vi "Autonomous Independent.vi"() -> ()   [LabVIEW 2013]
doc: "This VI is called when autonomous begins, and will automatically be terminated when autonomous ends. You can carry out timed or sensor driven robot movement independently without needing to return to the caller."
uses:
  Robot Global Data.vi
  <vilib>/addons/control/pid/pid.llb/PID (DBL).vi
  <vilib>/Rock Robotics/WPI/Joystick/WPI_JoystickGetSetRefNum.vi
  <vilib>/addons/control/pid/NI_PID_pid.lvlib
panel:
  out "Driver Station Digital Input (1-8)":bool[](array[boolean])
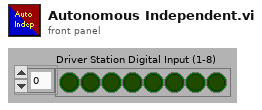
[diagram p1: front panel]
types:
  T1 = typedef "WPI_JoystickDevRef.ctl" = cluster{"Device":T2}
  T2 = typedef "WPI_JoystickDeviceEnum.ctl" = enum16{"USB 1", "USB 2", "USB 3", "USB 4", "Kinect 1", "Kinect 2"}
  T3 = cluster{"axis 1 (x)":dbl, "axis 2 (y)":dbl, "axis 3 (throttle)":dbl, "axis 4":dbl, "axis 5":dbl, "axis 6":dbl}
  T4 = cluster{"Driver Station Digital Input (1-8)[0]":bool, "Driver Station Digital Input (1-8)[1]":bool, "Driver Station Digital Input (1-8)[2]":bool, "Driver Station Digital Input (1-8)[3]":bool, "Driver Station Digital Input (1-8)[4]":bool, "Driver Station Digital Input (1-8)[5]":bool, "Driver Station Digital Input (1-8)[6]":bool, "Driver Station Digital Input (1-8)[7]":bool, "Driver Station Digital Input (1-8)[8]":bool}
  T5 = cluster{"proportional gain (Kc)":dbl, "integral time (Ti, min)":dbl, "derivative time (Td, min)":dbl}
  T6 = typedef "WPI_MotorControlDeviceRef.ctl" = cluster{"DeviceStatus":errorcluster, "Type":enum16{"PWM", "CAN"}, "PWM":cluster{"Digital Module":T7, "PWM Channel":T8, "DeadBand":T9}, "CAN":cluster{"Device Number":u8, "Control Mode":T10, "Semaphore":T11, "Max Vout":dbl}, "Invert":bool, "TransformRef":T12, "InvTransformRef":T12}
  T7 = typedef "FPGA_TypedefDigitalModule.ctl" = enum16{"Digital Module 1", "Digital Module 2"}
  T8 = typedef "FPGA_DIOPWMChannel.ctl" = enum8{"PWM 1", "PWM 2", "PWM 3", "PWM 4", "PWM 5", "PWM 6", "PWM 7", "PWM 8", "PWM 9", "PWM 10", "Invalid"}
  T9 = typedef "WPI_PWMDeadband.ctl" = cluster{"Name":string, "maxPositivePwm":i32, "minPositivePwm":i32, "centerPwm":i32, "maxNegativePwm":i32, "minNegativePwm":i32, "angularRange":u16}
  T10 = typedef "WPI_CANJaguar_ControlMode.ctl" = enum8{"Percent VBus", "Current", "Speed", "Position", "Voltage"}
  T11 = typedef "Semaphore RefNum" = refnum<k1>
  T12 = typedef "WPI_PWMTransform_ConPane.ctl" = refnum<vi>
  T13 = typedef "WPI_RobotDriveDevRef.ctl" = cluster{"DevStatus":errorcluster, "Motors[]":T6[], "Square Inputs":bool, "Max Output":dbl, "Isochronous":bool}
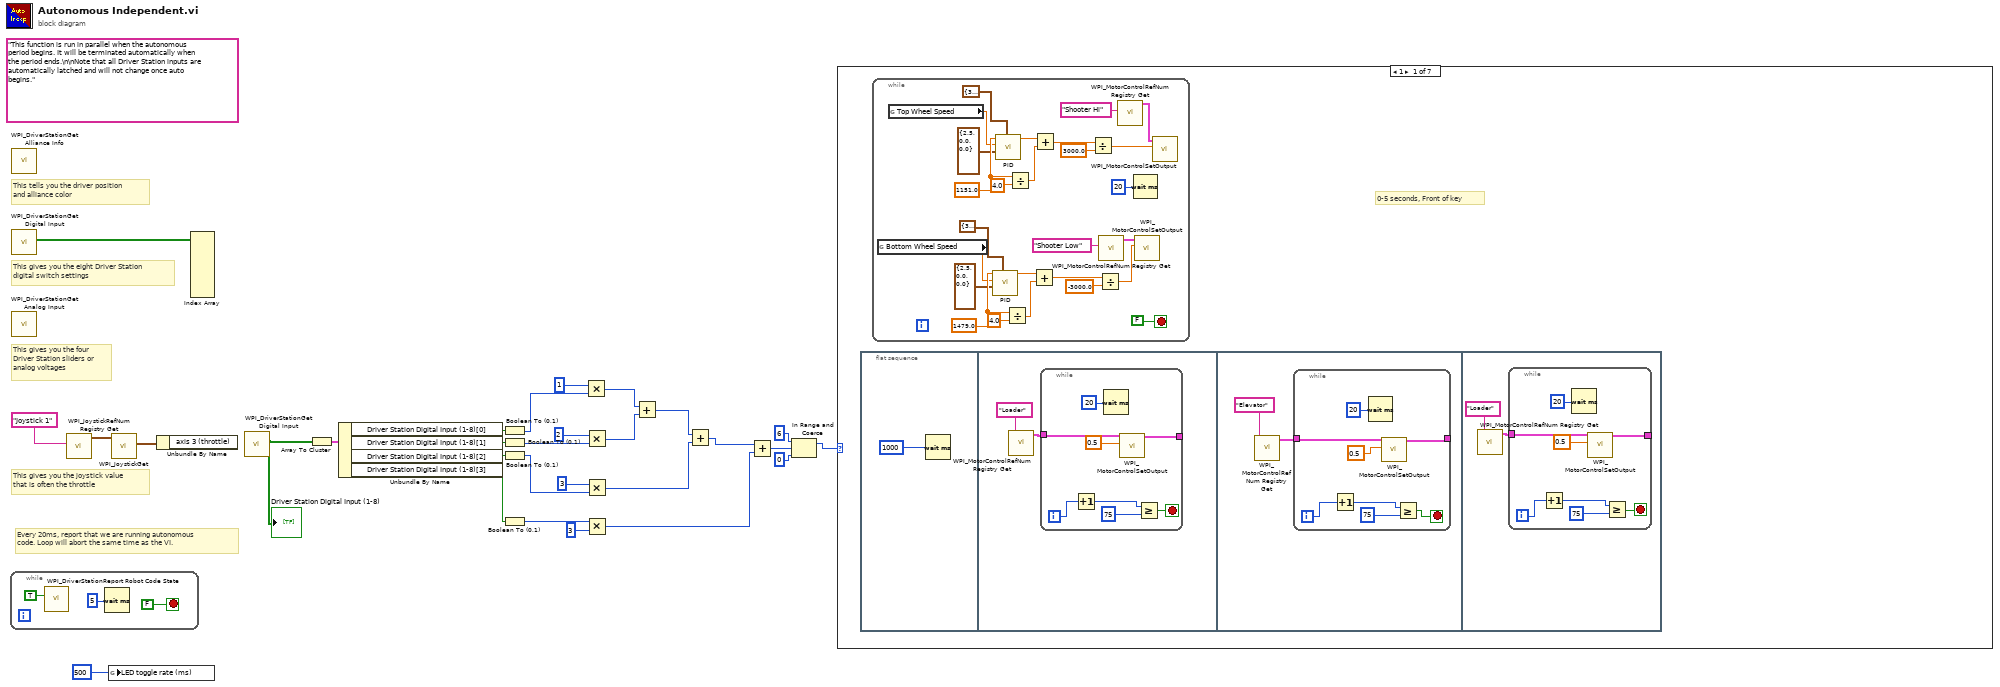
[diagram p0: block diagram]
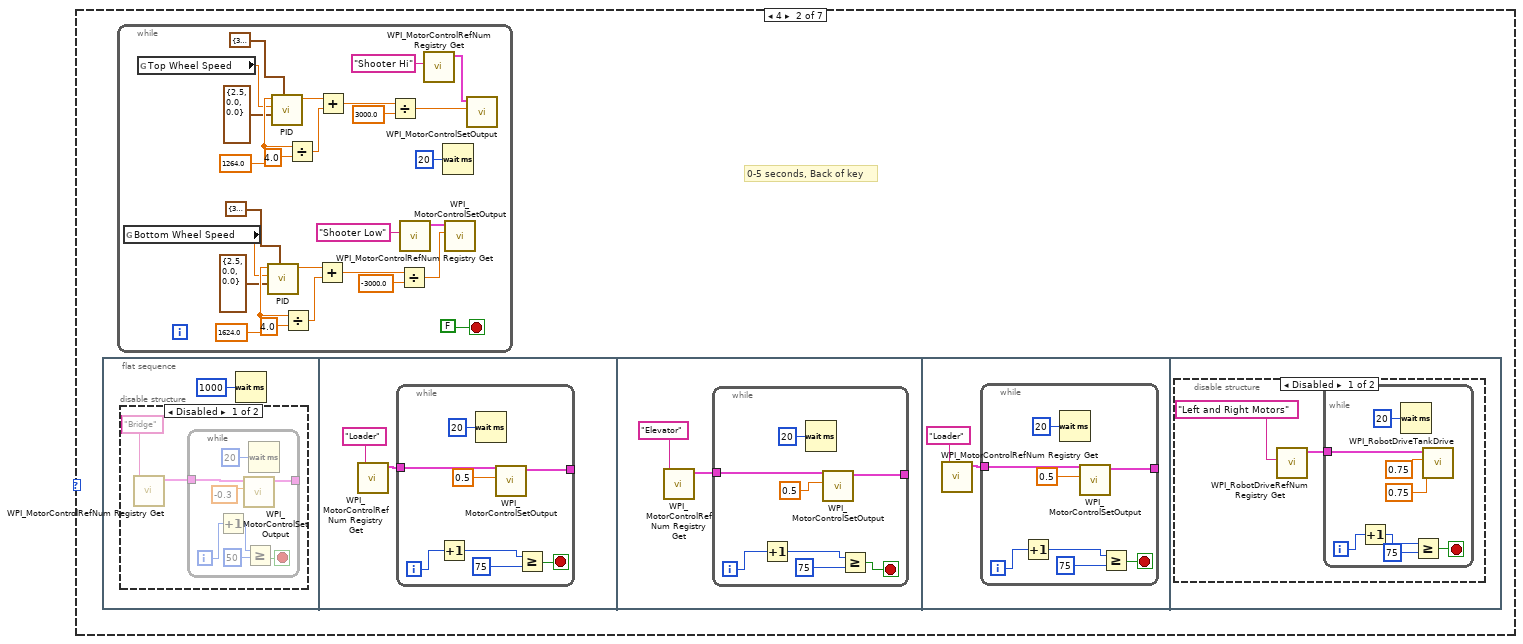
[diagram p2: hidden frame]
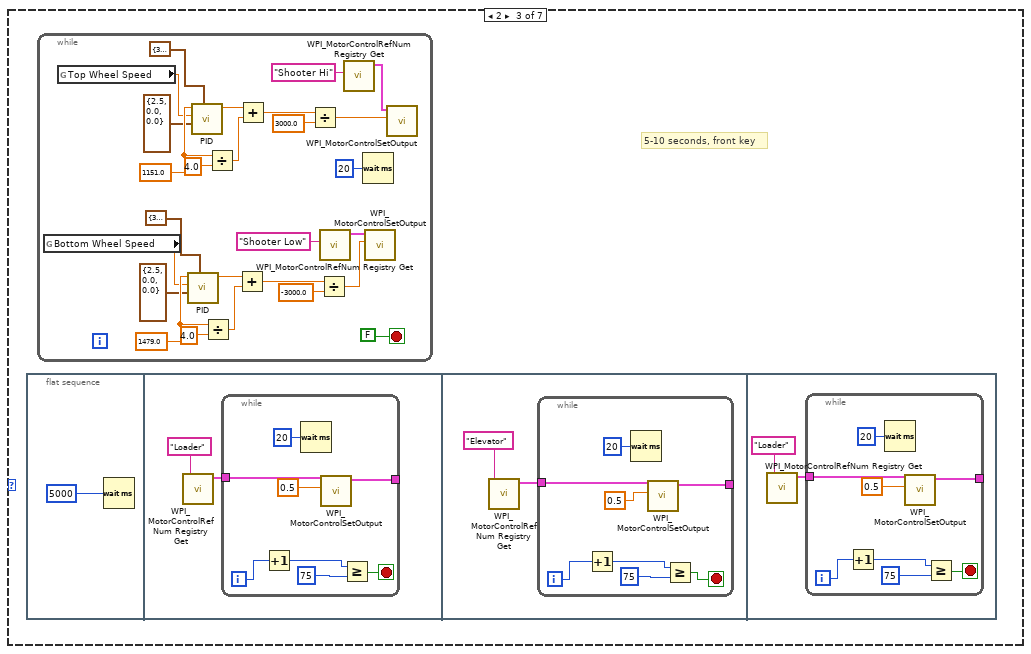
[diagram p5: hidden frame]
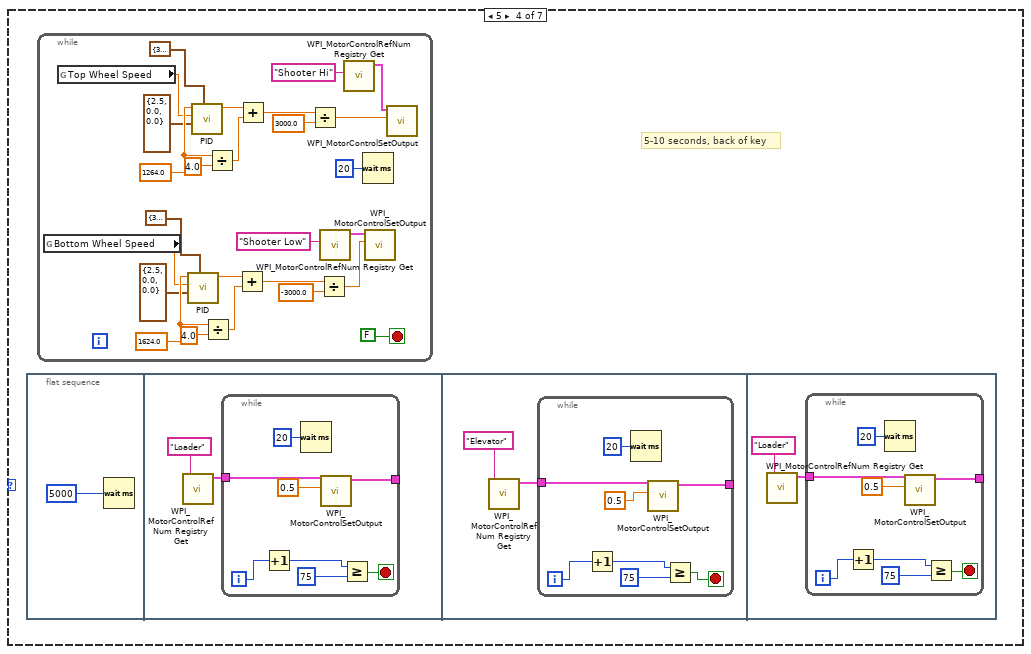
[diagram p6: hidden frame]
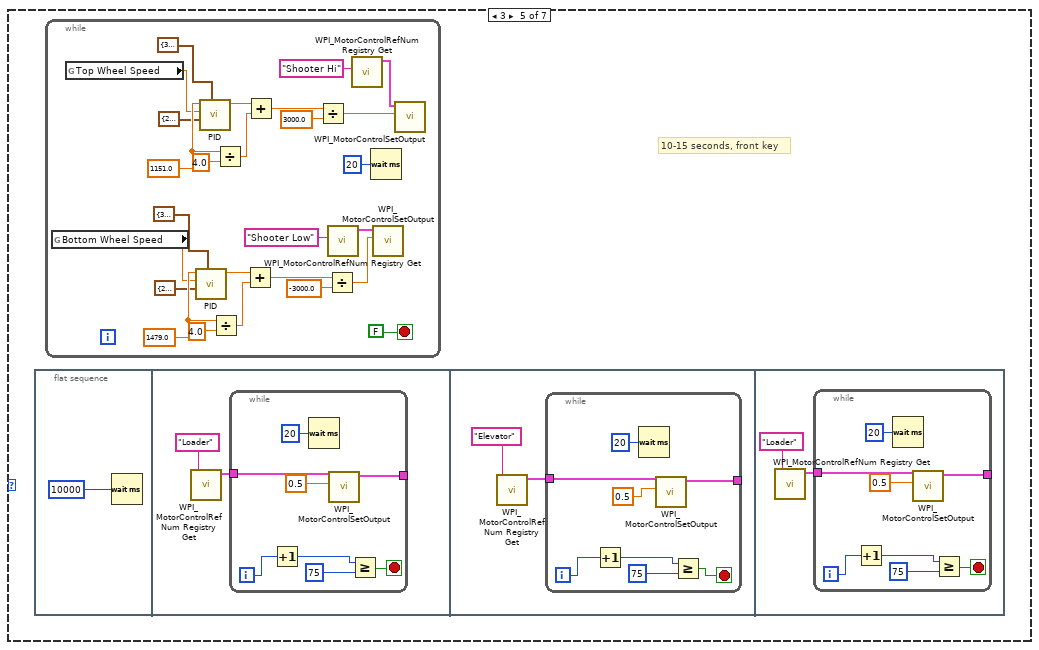
[diagram p7: hidden frame]
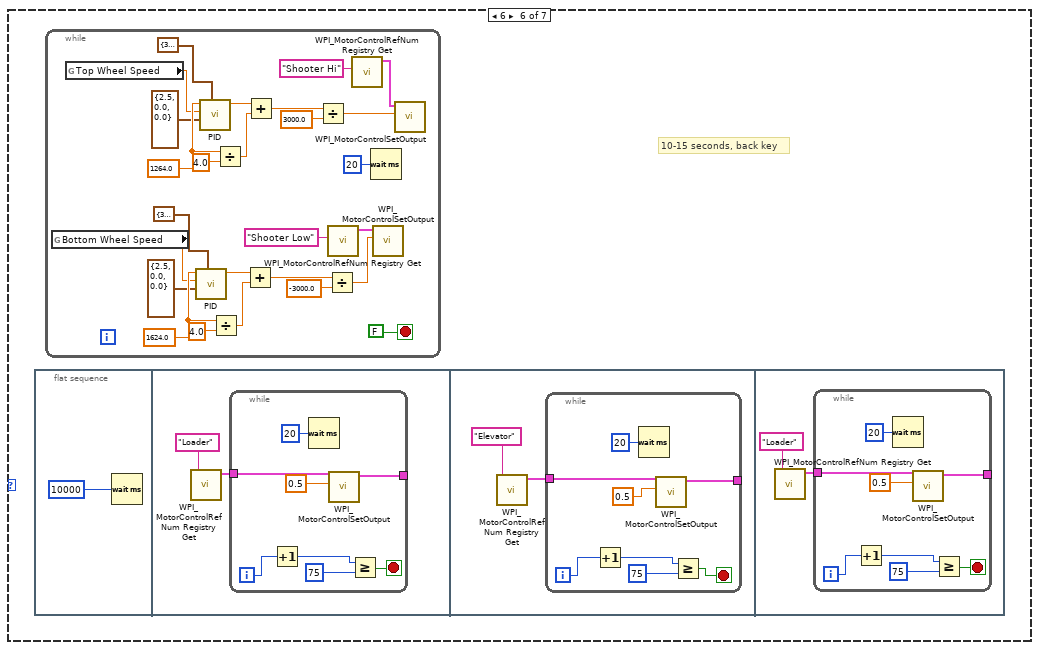
[diagram p8: hidden frame]
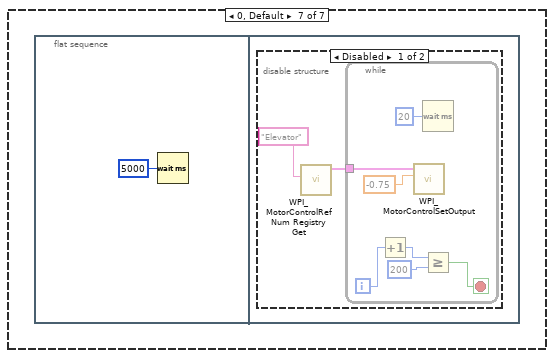
[diagram p9: hidden frame]
diagram:
  (unwired) "This function is run in parallel when the autonomous period begins. It will be terminated automatically when the period ends.\n\nNote that all Driver Station inputs are automatically latched and will not change once auto begins."
  # "Every 20ms, report that we are running autonomous\ncode. Loop will abort the same time as the VI."
  # "This gives you the joystick value\nthat is often the throttle"
  # "This tells you the driver position\nand alliance color"
  # "This gives you the eight Driver Station\ndigital switch settings"
  # "This gives you the four\nDriver Station sliders or\nanalog voltages"
  n1 = while {
    stop <- FALSE stop-if-true
    n2 = call <vilib>:"WPI_DriverStationReport Robot Code State.vi"("Autonomous"=TRUE) -> ()  [unwired: 10 in, 1 out]
    n3 = Wait (ms)(milliseconds to wait=u32 5) -> ()  [unwired: 1 out]
  }
  n4 = call <vilib>:"WPI_DriverStationGet Alliance Info.vi"() -> ()  [unwired: 12 out]
  n5 = call <vilib>:"WPI_DriverStationGet Digital Input.vi"() -> ("Driver Station Digital Input (1-8)"=w29:bool[])  [unwired: 11 out]
  n6 = call <vilib>:"WPI_DriverStationGet Analog Input.vi"() -> ()  [unwired: 12 out]
  n7 = call <vilib>:"WPI_JoystickRefNum Registry Get.vi"("refnum name"="Joystick 1") -> ("JoystickDevRef"=w26:T1)  [unwired: 1 in, 9 out]
  n8 = global write "Robot Global Data.vi" "LED toggle rate (ms)"(u32 500 ("LED ms toggle rate")) -> ()
  n9 = call <vilib>:"WPI_JoystickGet.vi"("JoystickDevRef"=w26) -> ("Axes"=w27:T3)  [unwired: 1 in, 5 out]
  n10 = Unbundle By Name(w27) -> ()  [unwired: 1 out]
  n11 = Index Array(array=w29) -> ()  [unwired: 8 in, 8 out]
  n12 = call <vilib>:"WPI_DriverStationGet Digital Input.vi"() -> ("Driver Station Digital Input (1-8)"=w24:bool[])  [unwired: 11 in]
  "Driver Station Digital Input (1-8)" <- w24
  n13 = Array To Cluster(array=w24) -> (cluster=w23:T4)
  n14 = Unbundle By Name(w23) -> ("Driver Station Digital Input (1-8)[0]"=w22:bool, "Driver Station Digital Input (1-8)[1]"=w21:bool, "Driver Station Digital Input (1-8)[2]"=w20:bool, "Driver Station Digital Input (1-8)[3]"=w9:bool)
  n15 = Boolean To (0,1)(Boolean=w22) -> (0, 1=w19:i16)
  n16 = Boolean To (0,1)(Boolean=w21) -> (0, 1=w18:i16)
  n17 = Boolean To (0,1)(Boolean=w20) -> (0, 1=w17:i16)
  n18 = Boolean To (0,1)(Boolean=w9) -> (0, 1=w8:i16)
  n19 = Multiply(x=1, y=w19) -> (x*y=w13:i32)
  n20 = Multiply(x=2, y=w18) -> (x*y=w12:i32)
  n21 = Multiply(x=3, y=w17) -> (x*y=w11:i32)
  n22 = Multiply(x=w8, y=i16 3) -> (x*y=w6:i16)
  n23 = Add(x=w13, y=w12) -> (x+y=w10:i32)
  n24 = Add(x=w10, y=w11) -> (x+y=w7:i32)
  n25 = Add(x=w7, y=w6) -> (x+y=w4:i32)
  n26 = In Range and Coerce(upper limit=6, x=w4, lower limit=0) -> (coerced(x)=w1:i32)  [unwired: 1 out]
  n27 = case shown="1" w1 {
    frame 1 {
      # "0-5 seconds, Front of key"
      n28 = flat-sequence {
        frame #0 {
          n29 = Wait (ms)(milliseconds to wait=u32 1000) -> ()  [unwired: 1 out]
        }
        frame #1 {
          n30 = call <vilib>:"WPI_MotorControlRefNum Registry Get.vi"("refnum name"="Loader") -> ("MotorControlDevRef"=w61:T6)  [unwired: 9 in, 1 out]
          n31 = while {
            tunnel: w61 -> [w69]
            tunnel: [w62] -> _
            i -> [w66]
            stop <- w63 stop-if-true
            n32 = Increment(x=w66) -> (x+1=w65:i32)
            n33 = Wait (ms)(milliseconds to wait=u32 20) -> ()  [unwired: 1 out]
            n34 = call <vilib>:"WPI_MotorControlSetOutput.vi"("Output"=0.5, "MotorControlDevRef"=w69) -> ("MotorControlDevRef"=w62:T6)  [unwired: 7 in, 2 out]
            n35 = Greater Or Equal?(x=w65, y=75) -> (x >= y?=w63:bool)
          }
        }
        frame #2 {
          n36 = call <vilib>:"WPI_MotorControlRefNum Registry Get.vi"("refnum name"="Elevator") -> ("MotorControlDevRef"=w71:T6)  [unwired: 9 in, 1 out]
          n37 = while {
            tunnel: w71 -> [w78]
            tunnel: [w72] -> _
            i -> [w74]
            stop <- w73 stop-if-true
            n38 = Increment(x=w74) -> (x+1=w76:i32)
            n39 = Wait (ms)(milliseconds to wait=u32 20) -> ()  [unwired: 1 out]
            n40 = call <vilib>:"WPI_MotorControlSetOutput.vi"("Output"=0.5, "MotorControlDevRef"=w78) -> ("MotorControlDevRef"=w72:T6)  [unwired: 7 in, 2 out]
            n41 = Greater Or Equal?(x=w76, y=75) -> (x >= y?=w73:bool)
          }
        }
        frame #3 {
          n42 = call <vilib>:"WPI_MotorControlRefNum Registry Get.vi"("refnum name"="Loader") -> ("MotorControlDevRef"=w81:T6)  [unwired: 9 in, 1 out]
          n43 = while {
            tunnel: w81 -> [w89]
            tunnel: [w82] -> _
            i -> [w86]
            stop <- w83 stop-if-true
            n44 = Increment(x=w86) -> (x+1=w85:i32)
            n45 = Wait (ms)(milliseconds to wait=u32 20) -> ()  [unwired: 1 out]
            n46 = call <vilib>:"WPI_MotorControlSetOutput.vi"("Output"=0.5, "MotorControlDevRef"=w89) -> ("MotorControlDevRef"=w82:T6)  [unwired: 7 in, 2 out]
            n47 = Greater Or Equal?(x=w85, y=75) -> (x >= y?=w83:bool)
          }
        }
      }
      n48 = while {
        stop <- FALSE stop-if-true
        w41 = 1479.0 ("setpoint")
        w49 = 1151.0 ("setpoint")
        n49 = global read "Robot Global Data.vi" "Bottom Wheel Speed"() -> (w40:dbl)
        n50 = global read "Robot Global Data.vi" "Top Wheel Speed"() -> (w47:dbl)
        n51 = call-poly <vilib>:"PID.vi"("output range"=cluster{"output high":dbl, "output low":dbl} {"output high"=3000.0, "output low"=0.0}, "PID gains"=T5 {"proportional gain (Kc)"=2.5, "integral time (Ti, min)"=0.0, "derivative time (Td, min)"=0.0}, "process variable"=w40, "setpoint"=w41) -> ("output"=w36:dbl)  [unwired: 6 in, 1 out]
        n52 = call-poly <vilib>:"PID.vi"("output range"=cluster{"output high":dbl, "output low":dbl} {"output high"=3000.0, "output low"=0.0}, "PID gains"=T5 {"proportional gain (Kc)"=2.5, "integral time (Ti, min)"=0.0, "derivative time (Td, min)"=0.0}, "process variable"=w47, "setpoint"=w49) -> ("output"=w43:dbl)  [unwired: 6 in, 1 out]
        n53 = Divide(x=w41, y=4.0) -> (x/y=w37:dbl)
        n54 = Divide(x=w49, y=4.0) -> (x/y=w44:dbl)
        n55 = Add(x=w36, y=w37) -> (x+y=w34:dbl)
        n56 = Add(x=w43, y=w44) -> (x+y=w42:dbl)
        n57 = Divide(x=w42, y=3000.0) -> (x/y=w51:dbl)
        n58 = Divide(x=w34, y=-3000.0) -> (x/y=w50:dbl)
        n59 = call <vilib>:"WPI_MotorControlRefNum Registry Get.vi"("refnum name"="Shooter Low") -> ("MotorControlDevRef"=w55:T6)  [unwired: 9 in, 1 out]
        n60 = call <vilib>:"WPI_MotorControlRefNum Registry Get.vi"("refnum name"="Shooter Hi") -> ("MotorControlDevRef"=w56:T6)  [unwired: 9 in, 1 out]
        n61 = Wait (ms)(milliseconds to wait=u32 20) -> ()  [unwired: 1 out]
        n62 = call <vilib>:"WPI_MotorControlSetOutput.vi"("Output"=w50, "MotorControlDevRef"=w55) -> ()  [unwired: 7 in, 3 out]
        n63 = call <vilib>:"WPI_MotorControlSetOutput.vi"("Output"=w51, "MotorControlDevRef"=w56) -> ()  [unwired: 7 in, 3 out]
      }
    }
    frame 4 {
      # "0-5 seconds, Back of key"
      n64 = flat-sequence {
        frame #0 {
          n65 = disable-structure shown="Disabled" {
            frame Disabled {
              n66 = call <vilib>:"WPI_MotorControlRefNum Registry Get.vi"("refnum name"="Bridge") -> ("MotorControlDevRef"=w117:T6)  [unwired: 9 in, 1 out]
              n67 = while {
                tunnel: w117 -> [w126]
                tunnel: [w125] -> _
                i -> [w122]
                stop <- w121 stop-if-true
                n68 = Increment(x=w122) -> (x+1=w120:i32)
                n69 = call <vilib>:"WPI_MotorControlSetOutput.vi"("Output"=-0.3, "MotorControlDevRef"=w126) -> ("MotorControlDevRef"=w125:T6)  [unwired: 7 in, 2 out]
                n70 = Greater Or Equal?(x=w120, y=50) -> (x >= y?=w121:bool)
                n71 = Wait (ms)(milliseconds to wait=u32 20) -> ()  [unwired: 1 out]
              }
            }
            frame Enabled {
            }
          }
          n72 = Wait (ms)(milliseconds to wait=u32 1000) -> ()  [unwired: 1 out]
        }
        frame #1 {
          n73 = call <vilib>:"WPI_MotorControlRefNum Registry Get.vi"("refnum name"="Loader") -> ("MotorControlDevRef"=w128:T6)  [unwired: 9 in, 1 out]
          n74 = while {
            tunnel: w128 -> [w136]
            tunnel: [w129] -> _
            i -> [w133]
            stop <- w130 stop-if-true
            n75 = Increment(x=w133) -> (x+1=w132:i32)
            n76 = Wait (ms)(milliseconds to wait=u32 20) -> ()  [unwired: 1 out]
            n77 = call <vilib>:"WPI_MotorControlSetOutput.vi"("Output"=0.5, "MotorControlDevRef"=w136) -> ("MotorControlDevRef"=w129:T6)  [unwired: 7 in, 2 out]
            n78 = Greater Or Equal?(x=w132, y=75) -> (x >= y?=w130:bool)
          }
        }
        frame #2 {
          n79 = call <vilib>:"WPI_MotorControlRefNum Registry Get.vi"("refnum name"="Elevator") -> ("MotorControlDevRef"=w138:T6)  [unwired: 9 in, 1 out]
          n80 = while {
            tunnel: w138 -> [w145]
            tunnel: [w139] -> _
            i -> [w141]
            stop <- w140 stop-if-true
            n81 = Increment(x=w141) -> (x+1=w143:i32)
            n82 = Wait (ms)(milliseconds to wait=u32 20) -> ()  [unwired: 1 out]
            n83 = call <vilib>:"WPI_MotorControlSetOutput.vi"("Output"=0.5, "MotorControlDevRef"=w145) -> ("MotorControlDevRef"=w139:T6)  [unwired: 7 in, 2 out]
            n84 = Greater Or Equal?(x=w143, y=75) -> (x >= y?=w140:bool)
          }
        }
        frame #3 {
          n85 = call <vilib>:"WPI_MotorControlRefNum Registry Get.vi"("refnum name"="Loader") -> ("MotorControlDevRef"=w148:T6)  [unwired: 9 in, 1 out]
          n86 = while {
            tunnel: w148 -> [w156]
            tunnel: [w149] -> _
            i -> [w153]
            stop <- w150 stop-if-true
            n87 = Increment(x=w153) -> (x+1=w152:i32)
            n88 = Wait (ms)(milliseconds to wait=u32 20) -> ()  [unwired: 1 out]
            n89 = call <vilib>:"WPI_MotorControlSetOutput.vi"("Output"=0.5, "MotorControlDevRef"=w156) -> ("MotorControlDevRef"=w149:T6)  [unwired: 7 in, 2 out]
            n90 = Greater Or Equal?(x=w152, y=75) -> (x >= y?=w150:bool)
          }
        }
        frame #4 {
          n91 = disable-structure shown="Disabled" {
            frame Disabled {
              n92 = call <vilib>:"WPI_RobotDriveRefNum Registry Get.vi"("refnum name"="Left and Right Motors") -> ("RobotDriveDevRef"=w157:T13)  [unwired: 9 in, 1 out]
              n93 = while {
                tunnel: w157 -> [w166]
                i -> [w162]
                stop <- w161 stop-if-true
                n94 = Increment(x=w162) -> (x+1=w160:i32)
                n95 = Wait (ms)(milliseconds to wait=u32 20) -> ()  [unwired: 1 out]
                n96 = Greater Or Equal?(x=w160, y=75) -> (x >= y?=w161:bool)
                n97 = call <vilib>:"WPI_RobotDriveTankDrive.vi"("Right axis value"=0.75, "Left axis value"=0.75, "RobotDriveDevRef"=w166) -> ()  [unwired: 6 in, 3 out]
              }
            }
            frame Enabled {
            }
          }
        }
      }
      n98 = while {
        stop <- FALSE stop-if-true
        w98 = 1624.0 ("setpoint")
        w106 = 1264.0 ("setpoint")
        n99 = global read "Robot Global Data.vi" "Bottom Wheel Speed"() -> (w97:dbl)
        n100 = global read "Robot Global Data.vi" "Top Wheel Speed"() -> (w104:dbl)
        n101 = call-poly <vilib>:"PID.vi"("output range"=cluster{"output high":dbl, "output low":dbl} {"output high"=3000.0, "output low"=0.0}, "PID gains"=T5 {"proportional gain (Kc)"=2.5, "integral time (Ti, min)"=0.0, "derivative time (Td, min)"=0.0}, "process variable"=w97, "setpoint"=w98) -> ("output"=w93:dbl)  [unwired: 6 in, 1 out]
        n102 = call-poly <vilib>:"PID.vi"("output range"=cluster{"output high":dbl, "output low":dbl} {"output high"=3000.0, "output low"=0.0}, "PID gains"=T5 {"proportional gain (Kc)"=2.5, "integral time (Ti, min)"=0.0, "derivative time (Td, min)"=0.0}, "process variable"=w104, "setpoint"=w106) -> ("output"=w100:dbl)  [unwired: 6 in, 1 out]
        n103 = Divide(x=w98, y=4.0) -> (x/y=w94:dbl)
        n104 = Divide(x=w106, y=4.0) -> (x/y=w101:dbl)
        n105 = Add(x=w93, y=w94) -> (x+y=w91:dbl)
        n106 = Add(x=w100, y=w101) -> (x+y=w99:dbl)
        n107 = Divide(x=w99, y=3000.0) -> (x/y=w108:dbl)
        n108 = Divide(x=w91, y=-3000.0) -> (x/y=w107:dbl)
        n109 = call <vilib>:"WPI_MotorControlRefNum Registry Get.vi"("refnum name"="Shooter Low") -> ("MotorControlDevRef"=w112:T6)  [unwired: 9 in, 1 out]
        n110 = call <vilib>:"WPI_MotorControlRefNum Registry Get.vi"("refnum name"="Shooter Hi") -> ("MotorControlDevRef"=w113:T6)  [unwired: 9 in, 1 out]
        n111 = Wait (ms)(milliseconds to wait=u32 20) -> ()  [unwired: 1 out]
        n112 = call <vilib>:"WPI_MotorControlSetOutput.vi"("Output"=w107, "MotorControlDevRef"=w112) -> ()  [unwired: 7 in, 3 out]
        n113 = call <vilib>:"WPI_MotorControlSetOutput.vi"("Output"=w108, "MotorControlDevRef"=w113) -> ()  [unwired: 7 in, 3 out]
      }
    }
    frame 2 {
      # "5-10 seconds, front key"
      n114 = flat-sequence {
        frame #0 {
          n115 = Wait (ms)(milliseconds to wait=u32 5000) -> ()  [unwired: 1 out]
        }
        frame #1 {
          n116 = call <vilib>:"WPI_MotorControlRefNum Registry Get.vi"("refnum name"="Loader") -> ("MotorControlDevRef"=w195:T6)  [unwired: 9 in, 1 out]
          n117 = while {
            tunnel: w195 -> [w203]
            tunnel: [w196] -> _
            i -> [w200]
            stop <- w197 stop-if-true
            n118 = Increment(x=w200) -> (x+1=w199:i32)
            n119 = Wait (ms)(milliseconds to wait=u32 20) -> ()  [unwired: 1 out]
            n120 = call <vilib>:"WPI_MotorControlSetOutput.vi"("Output"=0.5, "MotorControlDevRef"=w203) -> ("MotorControlDevRef"=w196:T6)  [unwired: 7 in, 2 out]
            n121 = Greater Or Equal?(x=w199, y=75) -> (x >= y?=w197:bool)
          }
        }
        frame #2 {
          n122 = call <vilib>:"WPI_MotorControlRefNum Registry Get.vi"("refnum name"="Elevator") -> ("MotorControlDevRef"=w205:T6)  [unwired: 9 in, 1 out]
          n123 = while {
            tunnel: w205 -> [w212]
            tunnel: [w206] -> _
            i -> [w208]
            stop <- w207 stop-if-true
            n124 = Increment(x=w208) -> (x+1=w210:i32)
            n125 = Wait (ms)(milliseconds to wait=u32 20) -> ()  [unwired: 1 out]
            n126 = call <vilib>:"WPI_MotorControlSetOutput.vi"("Output"=0.5, "MotorControlDevRef"=w212) -> ("MotorControlDevRef"=w206:T6)  [unwired: 7 in, 2 out]
            n127 = Greater Or Equal?(x=w210, y=75) -> (x >= y?=w207:bool)
          }
        }
        frame #3 {
          n128 = call <vilib>:"WPI_MotorControlRefNum Registry Get.vi"("refnum name"="Loader") -> ("MotorControlDevRef"=w215:T6)  [unwired: 9 in, 1 out]
          n129 = while {
            tunnel: w215 -> [w223]
            tunnel: [w216] -> _
            i -> [w220]
            stop <- w217 stop-if-true
            n130 = Increment(x=w220) -> (x+1=w219:i32)
            n131 = Wait (ms)(milliseconds to wait=u32 20) -> ()  [unwired: 1 out]
            n132 = call <vilib>:"WPI_MotorControlSetOutput.vi"("Output"=0.5, "MotorControlDevRef"=w223) -> ("MotorControlDevRef"=w216:T6)  [unwired: 7 in, 2 out]
            n133 = Greater Or Equal?(x=w219, y=75) -> (x >= y?=w217:bool)
          }
        }
      }
      n134 = while {
        stop <- FALSE stop-if-true
        w175 = 1479.0 ("setpoint")
        w183 = 1151.0 ("setpoint")
        n135 = global read "Robot Global Data.vi" "Bottom Wheel Speed"() -> (w174:dbl)
        n136 = global read "Robot Global Data.vi" "Top Wheel Speed"() -> (w181:dbl)
        n137 = call-poly <vilib>:"PID.vi"("output range"=cluster{"output high":dbl, "output low":dbl} {"output high"=3000.0, "output low"=0.0}, "PID gains"=T5 {"proportional gain (Kc)"=2.5, "integral time (Ti, min)"=0.0, "derivative time (Td, min)"=0.0}, "process variable"=w174, "setpoint"=w175) -> ("output"=w170:dbl)  [unwired: 6 in, 1 out]
        n138 = call-poly <vilib>:"PID.vi"("output range"=cluster{"output high":dbl, "output low":dbl} {"output high"=3000.0, "output low"=0.0}, "PID gains"=T5 {"proportional gain (Kc)"=2.5, "integral time (Ti, min)"=0.0, "derivative time (Td, min)"=0.0}, "process variable"=w181, "setpoint"=w183) -> ("output"=w177:dbl)  [unwired: 6 in, 1 out]
        n139 = Divide(x=w175, y=4.0) -> (x/y=w171:dbl)
        n140 = Divide(x=w183, y=4.0) -> (x/y=w178:dbl)
        n141 = Add(x=w170, y=w171) -> (x+y=w168:dbl)
        n142 = Add(x=w177, y=w178) -> (x+y=w176:dbl)
        n143 = Divide(x=w176, y=3000.0) -> (x/y=w185:dbl)
        n144 = Divide(x=w168, y=-3000.0) -> (x/y=w184:dbl)
        n145 = call <vilib>:"WPI_MotorControlRefNum Registry Get.vi"("refnum name"="Shooter Low") -> ("MotorControlDevRef"=w189:T6)  [unwired: 9 in, 1 out]
        n146 = call <vilib>:"WPI_MotorControlRefNum Registry Get.vi"("refnum name"="Shooter Hi") -> ("MotorControlDevRef"=w190:T6)  [unwired: 9 in, 1 out]
        n147 = Wait (ms)(milliseconds to wait=u32 20) -> ()  [unwired: 1 out]
        n148 = call <vilib>:"WPI_MotorControlSetOutput.vi"("Output"=w184, "MotorControlDevRef"=w189) -> ()  [unwired: 7 in, 3 out]
        n149 = call <vilib>:"WPI_MotorControlSetOutput.vi"("Output"=w185, "MotorControlDevRef"=w190) -> ()  [unwired: 7 in, 3 out]
      }
    }
    frame 5 {
      # "5-10 seconds, back of key"
      n150 = flat-sequence {
        frame #0 {
          n151 = Wait (ms)(milliseconds to wait=u32 5000) -> ()  [unwired: 1 out]
        }
        frame #1 {
          n152 = call <vilib>:"WPI_MotorControlRefNum Registry Get.vi"("refnum name"="Loader") -> ("MotorControlDevRef"=w252:T6)  [unwired: 9 in, 1 out]
          n153 = while {
            tunnel: w252 -> [w260]
            tunnel: [w253] -> _
            i -> [w257]
            stop <- w254 stop-if-true
            n154 = Increment(x=w257) -> (x+1=w256:i32)
            n155 = Wait (ms)(milliseconds to wait=u32 20) -> ()  [unwired: 1 out]
            n156 = call <vilib>:"WPI_MotorControlSetOutput.vi"("Output"=0.5, "MotorControlDevRef"=w260) -> ("MotorControlDevRef"=w253:T6)  [unwired: 7 in, 2 out]
            n157 = Greater Or Equal?(x=w256, y=75) -> (x >= y?=w254:bool)
          }
        }
        frame #2 {
          n158 = call <vilib>:"WPI_MotorControlRefNum Registry Get.vi"("refnum name"="Elevator") -> ("MotorControlDevRef"=w262:T6)  [unwired: 9 in, 1 out]
          n159 = while {
            tunnel: w262 -> [w269]
            tunnel: [w263] -> _
            i -> [w265]
            stop <- w264 stop-if-true
            n160 = Increment(x=w265) -> (x+1=w267:i32)
            n161 = Wait (ms)(milliseconds to wait=u32 20) -> ()  [unwired: 1 out]
            n162 = call <vilib>:"WPI_MotorControlSetOutput.vi"("Output"=0.5, "MotorControlDevRef"=w269) -> ("MotorControlDevRef"=w263:T6)  [unwired: 7 in, 2 out]
            n163 = Greater Or Equal?(x=w267, y=75) -> (x >= y?=w264:bool)
          }
        }
        frame #3 {
          n164 = call <vilib>:"WPI_MotorControlRefNum Registry Get.vi"("refnum name"="Loader") -> ("MotorControlDevRef"=w272:T6)  [unwired: 9 in, 1 out]
          n165 = while {
            tunnel: w272 -> [w280]
            tunnel: [w273] -> _
            i -> [w277]
            stop <- w274 stop-if-true
            n166 = Increment(x=w277) -> (x+1=w276:i32)
            n167 = Wait (ms)(milliseconds to wait=u32 20) -> ()  [unwired: 1 out]
            n168 = call <vilib>:"WPI_MotorControlSetOutput.vi"("Output"=0.5, "MotorControlDevRef"=w280) -> ("MotorControlDevRef"=w273:T6)  [unwired: 7 in, 2 out]
            n169 = Greater Or Equal?(x=w276, y=75) -> (x >= y?=w274:bool)
          }
        }
      }
      n170 = while {
        stop <- FALSE stop-if-true
        w232 = 1624.0 ("setpoint")
        w240 = 1264.0 ("setpoint")
        n171 = global read "Robot Global Data.vi" "Bottom Wheel Speed"() -> (w231:dbl)
        n172 = global read "Robot Global Data.vi" "Top Wheel Speed"() -> (w238:dbl)
        n173 = call-poly <vilib>:"PID.vi"("output range"=cluster{"output high":dbl, "output low":dbl} {"output high"=3000.0, "output low"=0.0}, "PID gains"=T5 {"proportional gain (Kc)"=2.5, "integral time (Ti, min)"=0.0, "derivative time (Td, min)"=0.0}, "process variable"=w231, "setpoint"=w232) -> ("output"=w227:dbl)  [unwired: 6 in, 1 out]
        n174 = call-poly <vilib>:"PID.vi"("output range"=cluster{"output high":dbl, "output low":dbl} {"output high"=3000.0, "output low"=0.0}, "PID gains"=T5 {"proportional gain (Kc)"=2.5, "integral time (Ti, min)"=0.0, "derivative time (Td, min)"=0.0}, "process variable"=w238, "setpoint"=w240) -> ("output"=w234:dbl)  [unwired: 6 in, 1 out]
        n175 = Divide(x=w232, y=4.0) -> (x/y=w228:dbl)
        n176 = Divide(x=w240, y=4.0) -> (x/y=w235:dbl)
        n177 = Add(x=w227, y=w228) -> (x+y=w225:dbl)
        n178 = Add(x=w234, y=w235) -> (x+y=w233:dbl)
        n179 = Divide(x=w233, y=3000.0) -> (x/y=w242:dbl)
        n180 = Divide(x=w225, y=-3000.0) -> (x/y=w241:dbl)
        n181 = call <vilib>:"WPI_MotorControlRefNum Registry Get.vi"("refnum name"="Shooter Low") -> ("MotorControlDevRef"=w246:T6)  [unwired: 9 in, 1 out]
        n182 = call <vilib>:"WPI_MotorControlRefNum Registry Get.vi"("refnum name"="Shooter Hi") -> ("MotorControlDevRef"=w247:T6)  [unwired: 9 in, 1 out]
        n183 = Wait (ms)(milliseconds to wait=u32 20) -> ()  [unwired: 1 out]
        n184 = call <vilib>:"WPI_MotorControlSetOutput.vi"("Output"=w241, "MotorControlDevRef"=w246) -> ()  [unwired: 7 in, 3 out]
        n185 = call <vilib>:"WPI_MotorControlSetOutput.vi"("Output"=w242, "MotorControlDevRef"=w247) -> ()  [unwired: 7 in, 3 out]
      }
    }
    frame 3 {
      # "10-15 seconds, front key"
      n186 = flat-sequence {
        frame #0 {
          n187 = Wait (ms)(milliseconds to wait=u32 10000) -> ()  [unwired: 1 out]
        }
        frame #1 {
          n188 = call <vilib>:"WPI_MotorControlRefNum Registry Get.vi"("refnum name"="Loader") -> ("MotorControlDevRef"=w309:T6)  [unwired: 9 in, 1 out]
          n189 = while {
            tunnel: w309 -> [w317]
            tunnel: [w310] -> _
            i -> [w314]
            stop <- w311 stop-if-true
            n190 = Increment(x=w314) -> (x+1=w313:i32)
            n191 = Wait (ms)(milliseconds to wait=u32 20) -> ()  [unwired: 1 out]
            n192 = call <vilib>:"WPI_MotorControlSetOutput.vi"("Output"=0.5, "MotorControlDevRef"=w317) -> ("MotorControlDevRef"=w310:T6)  [unwired: 7 in, 2 out]
            n193 = Greater Or Equal?(x=w313, y=75) -> (x >= y?=w311:bool)
          }
        }
        frame #2 {
          n194 = call <vilib>:"WPI_MotorControlRefNum Registry Get.vi"("refnum name"="Elevator") -> ("MotorControlDevRef"=w319:T6)  [unwired: 9 in, 1 out]
          n195 = while {
            tunnel: w319 -> [w326]
            tunnel: [w320] -> _
            i -> [w322]
            stop <- w321 stop-if-true
            n196 = Increment(x=w322) -> (x+1=w324:i32)
            n197 = Wait (ms)(milliseconds to wait=u32 20) -> ()  [unwired: 1 out]
            n198 = call <vilib>:"WPI_MotorControlSetOutput.vi"("Output"=0.5, "MotorControlDevRef"=w326) -> ("MotorControlDevRef"=w320:T6)  [unwired: 7 in, 2 out]
            n199 = Greater Or Equal?(x=w324, y=75) -> (x >= y?=w321:bool)
          }
        }
        frame #3 {
          n200 = call <vilib>:"WPI_MotorControlRefNum Registry Get.vi"("refnum name"="Loader") -> ("MotorControlDevRef"=w329:T6)  [unwired: 9 in, 1 out]
          n201 = while {
            tunnel: w329 -> [w337]
            tunnel: [w330] -> _
            i -> [w334]
            stop <- w331 stop-if-true
            n202 = Increment(x=w334) -> (x+1=w333:i32)
            n203 = Wait (ms)(milliseconds to wait=u32 20) -> ()  [unwired: 1 out]
            n204 = call <vilib>:"WPI_MotorControlSetOutput.vi"("Output"=0.5, "MotorControlDevRef"=w337) -> ("MotorControlDevRef"=w330:T6)  [unwired: 7 in, 2 out]
            n205 = Greater Or Equal?(x=w333, y=75) -> (x >= y?=w331:bool)
          }
        }
      }
      n206 = while {
        stop <- FALSE stop-if-true
        w289 = 1479.0 ("setpoint")
        w297 = 1151.0 ("setpoint")
        n207 = global read "Robot Global Data.vi" "Bottom Wheel Speed"() -> (w288:dbl)
        n208 = global read "Robot Global Data.vi" "Top Wheel Speed"() -> (w295:dbl)
        n209 = call-poly <vilib>:"PID.vi"("output range"=cluster{"output high":dbl, "output low":dbl} {"output high"=3000.0, "output low"=0.0}, "PID gains"=T5 {"proportional gain (Kc)"=2.5, "integral time (Ti, min)"=0.0, "derivative time (Td, min)"=0.0}, "process variable"=w288, "setpoint"=w289) -> ("output"=w284:dbl)  [unwired: 6 in, 1 out]
        n210 = call-poly <vilib>:"PID.vi"("output range"=cluster{"output high":dbl, "output low":dbl} {"output high"=3000.0, "output low"=0.0}, "PID gains"=T5 {"proportional gain (Kc)"=2.5, "integral time (Ti, min)"=0.0, "derivative time (Td, min)"=0.0}, "process variable"=w295, "setpoint"=w297) -> ("output"=w291:dbl)  [unwired: 6 in, 1 out]
        n211 = Divide(x=w289, y=4.0) -> (x/y=w285:dbl)
        n212 = Divide(x=w297, y=4.0) -> (x/y=w292:dbl)
        n213 = Add(x=w284, y=w285) -> (x+y=w282:dbl)
        n214 = Add(x=w291, y=w292) -> (x+y=w290:dbl)
        n215 = Divide(x=w290, y=3000.0) -> (x/y=w299:dbl)
        n216 = Divide(x=w282, y=-3000.0) -> (x/y=w298:dbl)
        n217 = call <vilib>:"WPI_MotorControlRefNum Registry Get.vi"("refnum name"="Shooter Low") -> ("MotorControlDevRef"=w303:T6)  [unwired: 9 in, 1 out]
        n218 = call <vilib>:"WPI_MotorControlRefNum Registry Get.vi"("refnum name"="Shooter Hi") -> ("MotorControlDevRef"=w304:T6)  [unwired: 9 in, 1 out]
        n219 = Wait (ms)(milliseconds to wait=u32 20) -> ()  [unwired: 1 out]
        n220 = call <vilib>:"WPI_MotorControlSetOutput.vi"("Output"=w298, "MotorControlDevRef"=w303) -> ()  [unwired: 7 in, 3 out]
        n221 = call <vilib>:"WPI_MotorControlSetOutput.vi"("Output"=w299, "MotorControlDevRef"=w304) -> ()  [unwired: 7 in, 3 out]
      }
    }
    frame 6 {
      # "10-15 seconds, back key"
      n222 = flat-sequence {
        frame #0 {
          n223 = Wait (ms)(milliseconds to wait=u32 10000) -> ()  [unwired: 1 out]
        }
        frame #1 {
          n224 = call <vilib>:"WPI_MotorControlRefNum Registry Get.vi"("refnum name"="Loader") -> ("MotorControlDevRef"=w366:T6)  [unwired: 9 in, 1 out]
          n225 = while {
            tunnel: w366 -> [w374]
            tunnel: [w367] -> _
            i -> [w371]
            stop <- w368 stop-if-true
            n226 = Increment(x=w371) -> (x+1=w370:i32)
            n227 = Wait (ms)(milliseconds to wait=u32 20) -> ()  [unwired: 1 out]
            n228 = call <vilib>:"WPI_MotorControlSetOutput.vi"("Output"=0.5, "MotorControlDevRef"=w374) -> ("MotorControlDevRef"=w367:T6)  [unwired: 7 in, 2 out]
            n229 = Greater Or Equal?(x=w370, y=75) -> (x >= y?=w368:bool)
          }
        }
        frame #2 {
          n230 = call <vilib>:"WPI_MotorControlRefNum Registry Get.vi"("refnum name"="Elevator") -> ("MotorControlDevRef"=w376:T6)  [unwired: 9 in, 1 out]
          n231 = while {
            tunnel: w376 -> [w383]
            tunnel: [w377] -> _
            i -> [w379]
            stop <- w378 stop-if-true
            n232 = Increment(x=w379) -> (x+1=w381:i32)
            n233 = Wait (ms)(milliseconds to wait=u32 20) -> ()  [unwired: 1 out]
            n234 = call <vilib>:"WPI_MotorControlSetOutput.vi"("Output"=0.5, "MotorControlDevRef"=w383) -> ("MotorControlDevRef"=w377:T6)  [unwired: 7 in, 2 out]
            n235 = Greater Or Equal?(x=w381, y=75) -> (x >= y?=w378:bool)
          }
        }
        frame #3 {
          n236 = call <vilib>:"WPI_MotorControlRefNum Registry Get.vi"("refnum name"="Loader") -> ("MotorControlDevRef"=w386:T6)  [unwired: 9 in, 1 out]
          n237 = while {
            tunnel: w386 -> [w394]
            tunnel: [w387] -> _
            i -> [w391]
            stop <- w388 stop-if-true
            n238 = Increment(x=w391) -> (x+1=w390:i32)
            n239 = Wait (ms)(milliseconds to wait=u32 20) -> ()  [unwired: 1 out]
            n240 = call <vilib>:"WPI_MotorControlSetOutput.vi"("Output"=0.5, "MotorControlDevRef"=w394) -> ("MotorControlDevRef"=w387:T6)  [unwired: 7 in, 2 out]
            n241 = Greater Or Equal?(x=w390, y=75) -> (x >= y?=w388:bool)
          }
        }
      }
      n242 = while {
        stop <- FALSE stop-if-true
        w346 = 1624.0 ("setpoint")
        w354 = 1264.0 ("setpoint")
        n243 = global read "Robot Global Data.vi" "Bottom Wheel Speed"() -> (w345:dbl)
        n244 = global read "Robot Global Data.vi" "Top Wheel Speed"() -> (w352:dbl)
        n245 = call-poly <vilib>:"PID.vi"("output range"=cluster{"output high":dbl, "output low":dbl} {"output high"=3000.0, "output low"=0.0}, "PID gains"=T5 {"proportional gain (Kc)"=2.5, "integral time (Ti, min)"=0.0, "derivative time (Td, min)"=0.0}, "process variable"=w345, "setpoint"=w346) -> ("output"=w341:dbl)  [unwired: 6 in, 1 out]
        n246 = call-poly <vilib>:"PID.vi"("output range"=cluster{"output high":dbl, "output low":dbl} {"output high"=3000.0, "output low"=0.0}, "PID gains"=T5 {"proportional gain (Kc)"=2.5, "integral time (Ti, min)"=0.0, "derivative time (Td, min)"=0.0}, "process variable"=w352, "setpoint"=w354) -> ("output"=w348:dbl)  [unwired: 6 in, 1 out]
        n247 = Divide(x=w346, y=4.0) -> (x/y=w342:dbl)
        n248 = Divide(x=w354, y=4.0) -> (x/y=w349:dbl)
        n249 = Add(x=w341, y=w342) -> (x+y=w339:dbl)
        n250 = Add(x=w348, y=w349) -> (x+y=w347:dbl)
        n251 = Divide(x=w347, y=3000.0) -> (x/y=w356:dbl)
        n252 = Divide(x=w339, y=-3000.0) -> (x/y=w355:dbl)
        n253 = call <vilib>:"WPI_MotorControlRefNum Registry Get.vi"("refnum name"="Shooter Low") -> ("MotorControlDevRef"=w360:T6)  [unwired: 9 in, 1 out]
        n254 = call <vilib>:"WPI_MotorControlRefNum Registry Get.vi"("refnum name"="Shooter Hi") -> ("MotorControlDevRef"=w361:T6)  [unwired: 9 in, 1 out]
        n255 = Wait (ms)(milliseconds to wait=u32 20) -> ()  [unwired: 1 out]
        n256 = call <vilib>:"WPI_MotorControlSetOutput.vi"("Output"=w355, "MotorControlDevRef"=w360) -> ()  [unwired: 7 in, 3 out]
        n257 = call <vilib>:"WPI_MotorControlSetOutput.vi"("Output"=w356, "MotorControlDevRef"=w361) -> ()  [unwired: 7 in, 3 out]
      }
    }
    frame 0, Default {
      n258 = flat-sequence {
        frame #0 {
          n259 = Wait (ms)(milliseconds to wait=u32 5000) -> ()  [unwired: 1 out]
        }
        frame #1 {
          n260 = disable-structure shown="Disabled" {
            frame Disabled {
              n261 = call <vilib>:"WPI_MotorControlRefNum Registry Get.vi"("refnum name"="Elevator") -> ("MotorControlDevRef"=w396:T6)  [unwired: 9 in, 1 out]
              n262 = while {
                tunnel: w396 -> [w404]
                i -> [w401]
                stop <- w398 stop-if-true
                n263 = Increment(x=w401) -> (x+1=w400:i32)
                n264 = call <vilib>:"WPI_MotorControlSetOutput.vi"("Output"=-0.75, "MotorControlDevRef"=w404) -> ()  [unwired: 7 in, 3 out]
                n265 = Wait (ms)(milliseconds to wait=u32 20) -> ()  [unwired: 1 out]
                n266 = Greater Or Equal?(x=w400, y=200) -> (x >= y?=w398:bool)
              }
            }
            frame Enabled {
            }
          }
        }
      }
    }
  }
